vi "Read Name.vi"(11 "ITem in":refnum<class "ITem.lvclass">) -> (3 "Name":string)   [LabVIEW 2020, in "ITem.lvclass"]
uses:
  ITem.lvclass
  ITem.lvclass/ITem.ctl
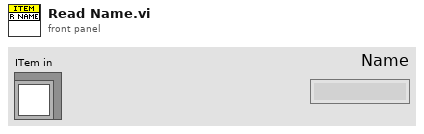
[diagram p1: front panel]
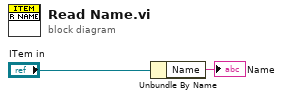
[diagram p0: block diagram]
diagram:
  n1 = Unbundle By Name("ITem in") -> ("Name"=→"Name":string)
